vi "LaserAutoShutter.vi"(7 "error in (no error)":errorcluster, 10 "reference In":refnum<k24>) -> (0 "error out":errorcluster, 3 "reference out":refnum<k24>)   [LabVIEW 2019]
doc: "Generates sample waveforms according to the signal type in the HW Config input."
uses:
  E:/DevHardSoftware/MMicroscopy/HardwareAdapter/Lasers/Dependencies/Oxxius_Boxx.dll
  Dependencies/Oxxius_Boxx.dll
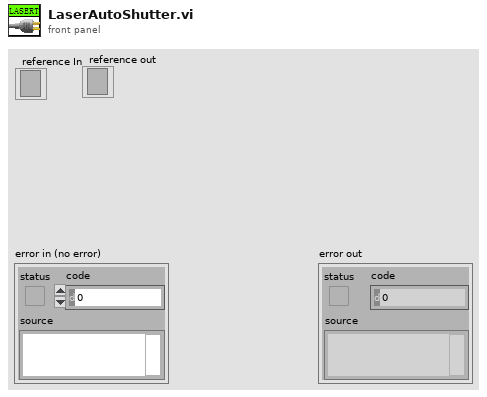
[diagram p1: front panel]
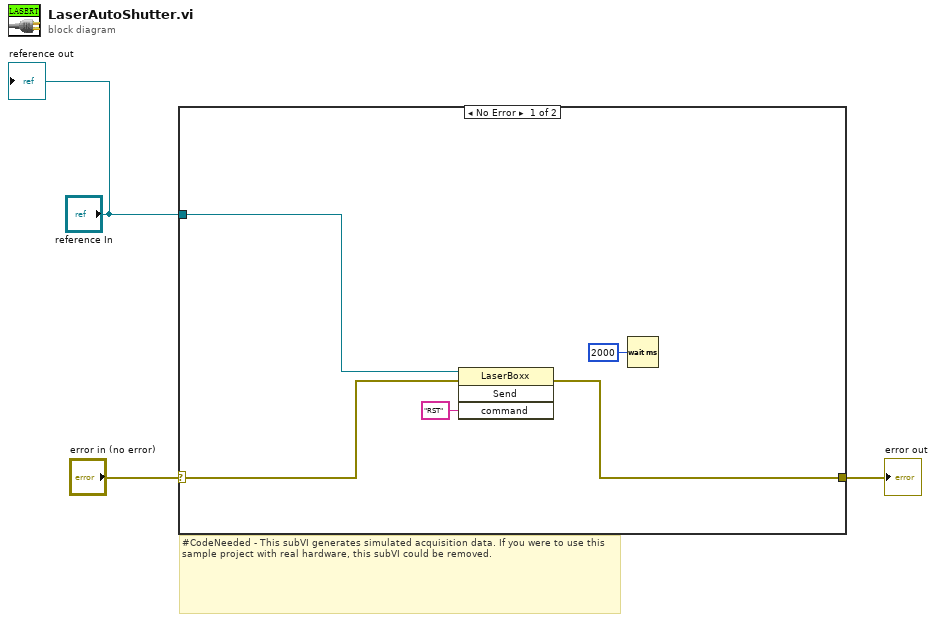
[diagram p0: block diagram]
diagram:
  # "#CodeNeeded - This subVI generates simulated acquisition data. If you were to use this sample project with real hardware, this subVI could be removed."
  n1 = case shown="No Error" "error in (no error)" {
    selector: "error in (no error)" -> [w7 w9]
    tunnel: [w8 w9] -> w2
    tunnel: "reference In" -> [w6 _]
    frame No Error {
      n2 = invoke class="LaserBoxx" method="Send"(reference=w6, error in=w7, "command"="RST") -> (error out=w8:errorcluster)  [unwired: 1 in, 3 out]
      n3 = Wait (ms)(milliseconds to wait=u32 2000) -> ()  [unwired: 1 out]
    }
    frame Error {
    }
  }
  "error out" <- w2
  "reference out" <- "reference In"
